vi "check_comfirm.vi"(3 "Choose movie":i32, 5 "NOC":i32, 6 "No. of seats":i32, 7 "Price":i32, 8 "Username":string, 9 "member":bool, 10 "Seats no.":i32[](array[numeric])) -> (0 "finish check":bool, 1 "Next state":T1(ring), 2 "TA":dbl, 4 "Leave":bool)   [LabVIEW 2014]
panel:
  in  "Cluster":cluster{"OK Button":bool, "OK Button 2":bool}
  out "Booking info":string
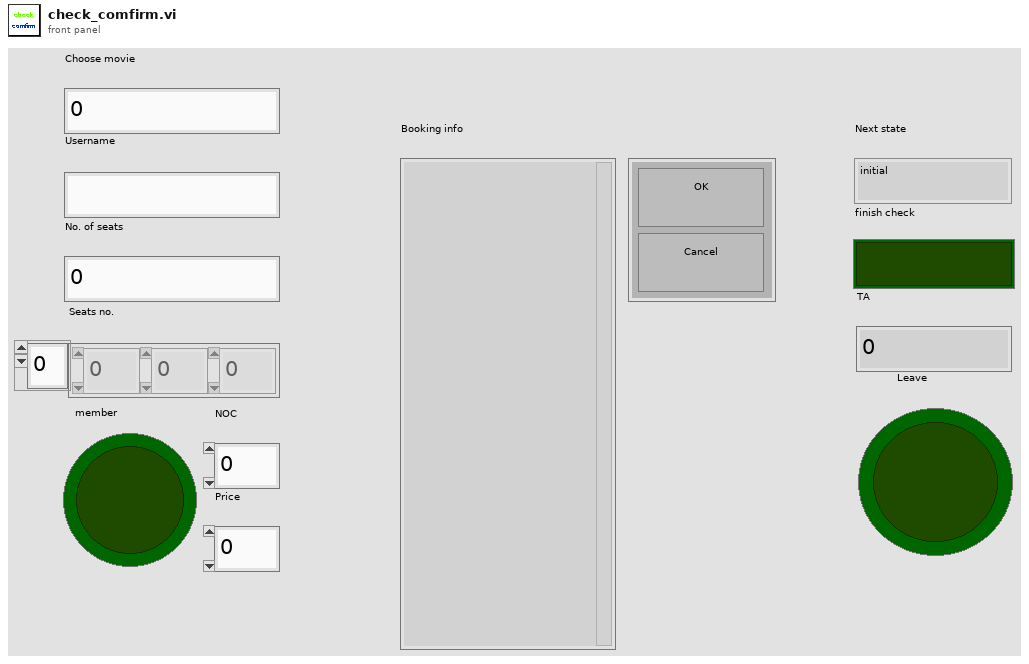
[diagram p1: front panel]
types:
  T1 = enum16{"initial", "start", "member?", "register?", "member login", "member register", "choose movie", "how many seat?", "check", "end"}
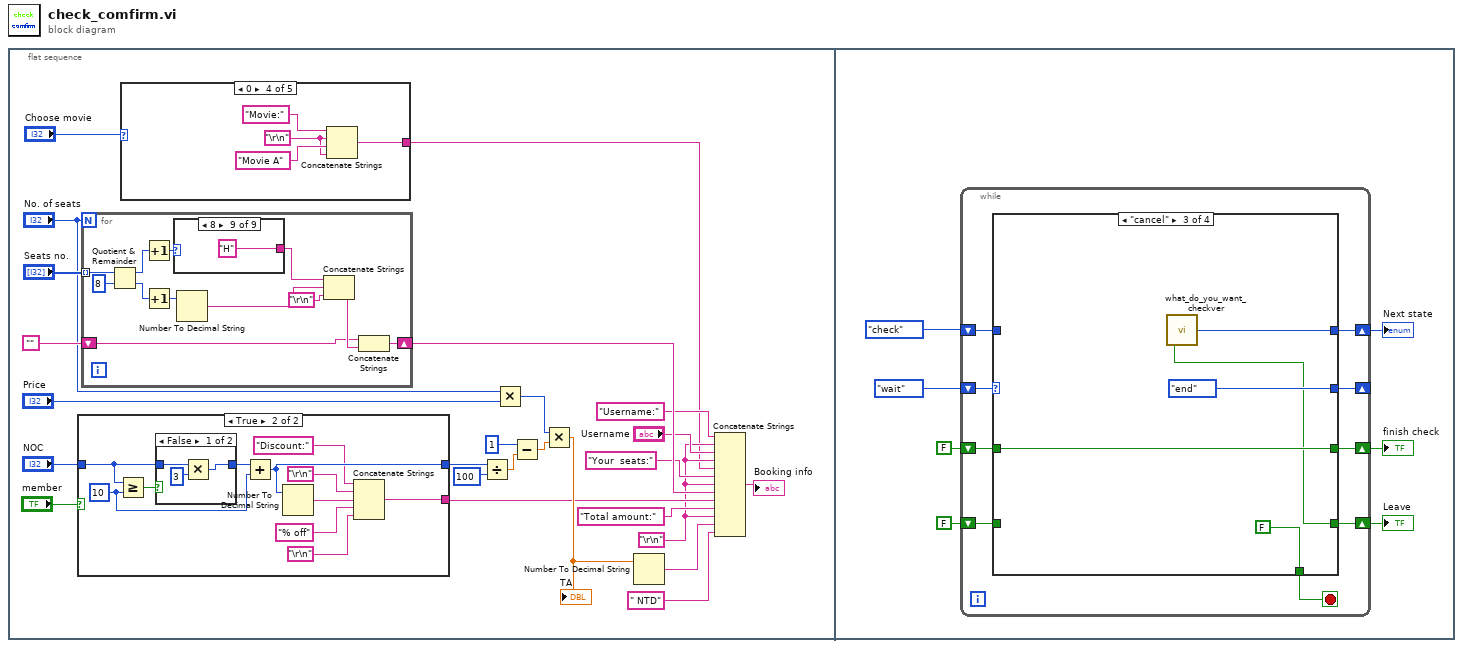
[diagram p0: block diagram]
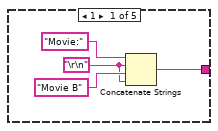
[diagram p2: hidden frame]
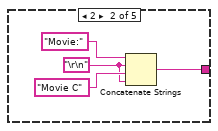
[diagram p3: hidden frame]
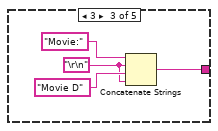
[diagram p4: hidden frame]
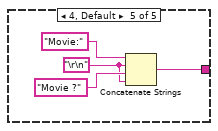
[diagram p5: hidden frame]
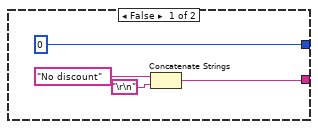
[diagram p6: hidden frame]
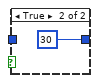
[diagram p7: hidden frame]
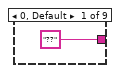
[diagram p8: hidden frame]
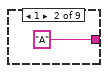
[diagram p9: hidden frame]
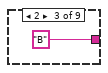
[diagram p10: hidden frame]
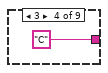
[diagram p11: hidden frame]
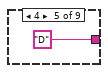
[diagram p12: hidden frame]
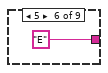
[diagram p13: hidden frame]
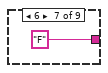
[diagram p14: hidden frame]
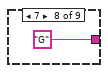
[diagram p15: hidden frame]
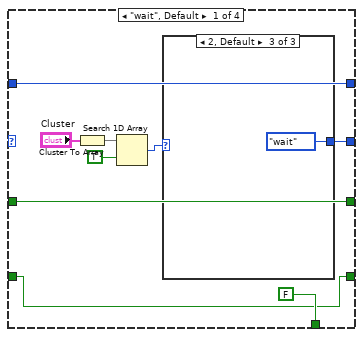
[diagram p16: hidden frame]
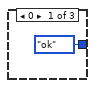
[diagram p17: hidden frame]
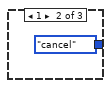
[diagram p18: hidden frame]
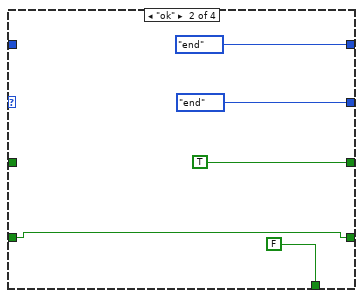
[diagram p19: hidden frame]
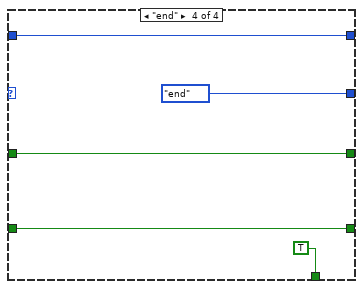
[diagram p20: hidden frame]
diagram:
  n1 = flat-sequence {
    frame #0 {
      w2 = "\r\n"
      n2 = case shown="True" "member" {
        tunnel: "NOC" -> [_ w59]
        tunnel: [0 w56] -> w21
        tunnel: [w46 w50] -> w10
        frame False {
          n3 = Concatenate Strings("No discount", "\r\n") -> (w46:string)
        }
        frame True {
          w57 = 10 ("y")
          n4 = Greater Or Equal?(x=w59, y=w57) -> (x >= y?=w60:bool)
          n5 = case shown="False" w60 {
            tunnel: w59 -> [w63 _]
            tunnel: [w61 30] -> w58
            frame False {
              n6 = Multiply(x=w63, y=3) -> (x*y=w61:i32)
            }
            frame True {
            }
          }
          n7 = Add(x=w58, y=w57) -> (x+y=w56:i32)
          n8 = Number To Decimal String(number=w56) -> (decimal integer string=w53:string)  [unwired: 1 in]
          n9 = Concatenate Strings("Discount:", "\r\n", w53, "% off", "\r\n") -> (w50:string)
        }
      }
      n10 = for {
        N: "No. of seats" -> [_]
        tunnel: "Seats no." -> [w76] mode=indexing
        shift-right: [w67] -> w9
        shift-left: "" -> [w65]
        n11 = Quotient & Remainder(x=w76, y=8) -> (x-y*floor(x/y)=w74:i32, floor(x/y)=w72:i32)
        n12 = Increment(x=w74) -> (x+1=w73:i32)
        n13 = Increment(x=w72) -> (x+1=w68:i32)
        n14 = case shown="8" w73 {
          tunnel: ["??" "A" "B" "C" "D" "E" "F" "G" "H"] -> w71
          frame 0, Default {
          }
          frame 1 {
          }
          frame 2 {
          }
          frame 3 {
          }
          frame 4 {
          }
          frame 5 {
          }
          frame 6 {
          }
          frame 7 {
          }
          frame 8 {
          }
        }
        n15 = Number To Decimal String(number=w68) -> (decimal integer string=w70:string)  [unwired: 1 in]
        n16 = Concatenate Strings(w71, w70, "\r\n") -> (w66:string)
        n17 = Concatenate Strings(w65, w66) -> (w67:string)
      }
      n18 = case shown="0" "Choose movie" {
        tunnel: [w26 w30 w34 w38 w42] -> w1
        frame 1 {
          w27 = "\r\n"
          n19 = Concatenate Strings("Movie:", w27, "Movie B", w27) -> (w26:string)
        }
        frame 2 {
          w31 = "\r\n"
          n20 = Concatenate Strings("Movie:", w31, "Movie C", w31) -> (w30:string)
        }
        frame 3 {
          w35 = "\r\n"
          n21 = Concatenate Strings("Movie:", w35, "Movie D", w35) -> (w34:string)
        }
        frame 0 {
          w39 = "\r\n"
          n22 = Concatenate Strings("Movie:", w39, "Movie A", w39) -> (w38:string)
        }
        frame 4, Default {
          w43 = "\r\n"
          n23 = Concatenate Strings("Movie:", w43, "Movie ?", w43) -> (w42:string)
        }
      }
      n24 = Divide(x=w21, y=100) -> (x/y=w19:dbl)
      n25 = Multiply(x="No. of seats", y="Price") -> (x*y=w16:i32)
      n26 = Subtract(x=1, y=w19) -> (x-y=w17:dbl)
      n27 = Multiply(x=w16, y=w17) -> (x*y=w13:dbl)
      "TA" <- w13
      n28 = Number To Decimal String(number=w13) -> (decimal integer string=w12:string)  [unwired: 1 in]
      n29 = Concatenate Strings("Username:", w2, "Username", w2, w1, "Your  seats:", w2, w9, w10, "Total amount:", w2, w12, " NTD") -> (→"Booking info":string)
    }
    frame #1 {
      n30 = while {
        shift-right: [w100] -> _
        shift-left: enum16{"wait", "ok", "cancel", "end"}."wait" -> [w101]
        shift-right: [w99] -> w90
        shift-left: T1."check" -> [w98]
        shift-right: [w96] -> w89
        shift-left: FALSE -> [w95]
        shift-right: [w94] -> w86
        shift-left: FALSE ("Leave") -> [w93]
        stop <- w97 stop-if-true
        n31 = case shown="\"cancel\"" w101 {
          tunnel: [w106 enum16{"wait", "ok", "cancel", "end"}."end" enum16{"wait", "ok", "cancel", "end"}."end" enum16{"wait", "ok", "cancel", "end"}."end"] -> w100
          tunnel: [w105 T1."end" w122 w127] -> w99
          tunnel: w98 -> [w105 _ _ w127]
          tunnel: [FALSE FALSE FALSE TRUE] -> w97
          tunnel: [w103 TRUE w120 w125] -> w96
          tunnel: w95 -> [w103 _ w120 w125]
          tunnel: [w102 w114 w119 w124] -> w94
          tunnel: w93 -> [w102 w114 _ w124]
          frame "wait", Default {
            n32 = Cluster To Array(cluster="Cluster") -> (array=w109:bool[])
            n33 = Search 1D Array(1D array=w109, element=TRUE) -> (index of element=w107:i32)  [unwired: 1 in]
            n34 = case shown="2, Default" w107 {
              tunnel: [enum16{"wait", "ok", "cancel", "end"}."ok" enum16{"wait", "ok", "cancel", "end"}."cancel" enum16{"wait", "ok", "cancel", "end"}."wait"] -> w106
              frame 0 {
              }
              frame 1 {
              }
              frame 2, Default {
              }
            }
          }
          frame "ok" {
          }
          frame "cancel" {
            n35 = call "what_do_you_want_checkver.vi"() -> ("Next state"=w122:T1, "Leave"=w119:bool)
          }
          frame "end" {
          }
        }
      }
      "Next state" <- w90
      "finish check" <- w89
      "Leave" <- w86
    }
  }
